vi "loadSRMSummary.vi"(7 "Machine":string, 10 "file path (dialog if empty)":path=path "C:/temp/SRM/S141201869.txt") -> (0 "error out":errorcluster)   [LabVIEW 2012]
uses:
  <vilib>/addons/database/Auxilliary.llb/DB Tools Cursor Type.ctl
  <vilib>/addons/database/Connection.llb/DB Tools Open Connec (Path).vi
  <vilib>/addons/database/Connection.llb/Conn Execute.vi
  <vilib>/addons/database/Recordset.llb/Rec Fetch Integer Data (R).vi
  <vilib>/addons/database/Recordset.llb/Rec Destroy - Connection.vi
  <vilib>/addons/database/NI_Database_API.lvlib
panel:
  out "after substring 2":string
  out "after substring":string
  in  "Cluster 2":T1
  out "array":string[][](array[string])
  out "concatenated string":string
  in  "Cluster":T2
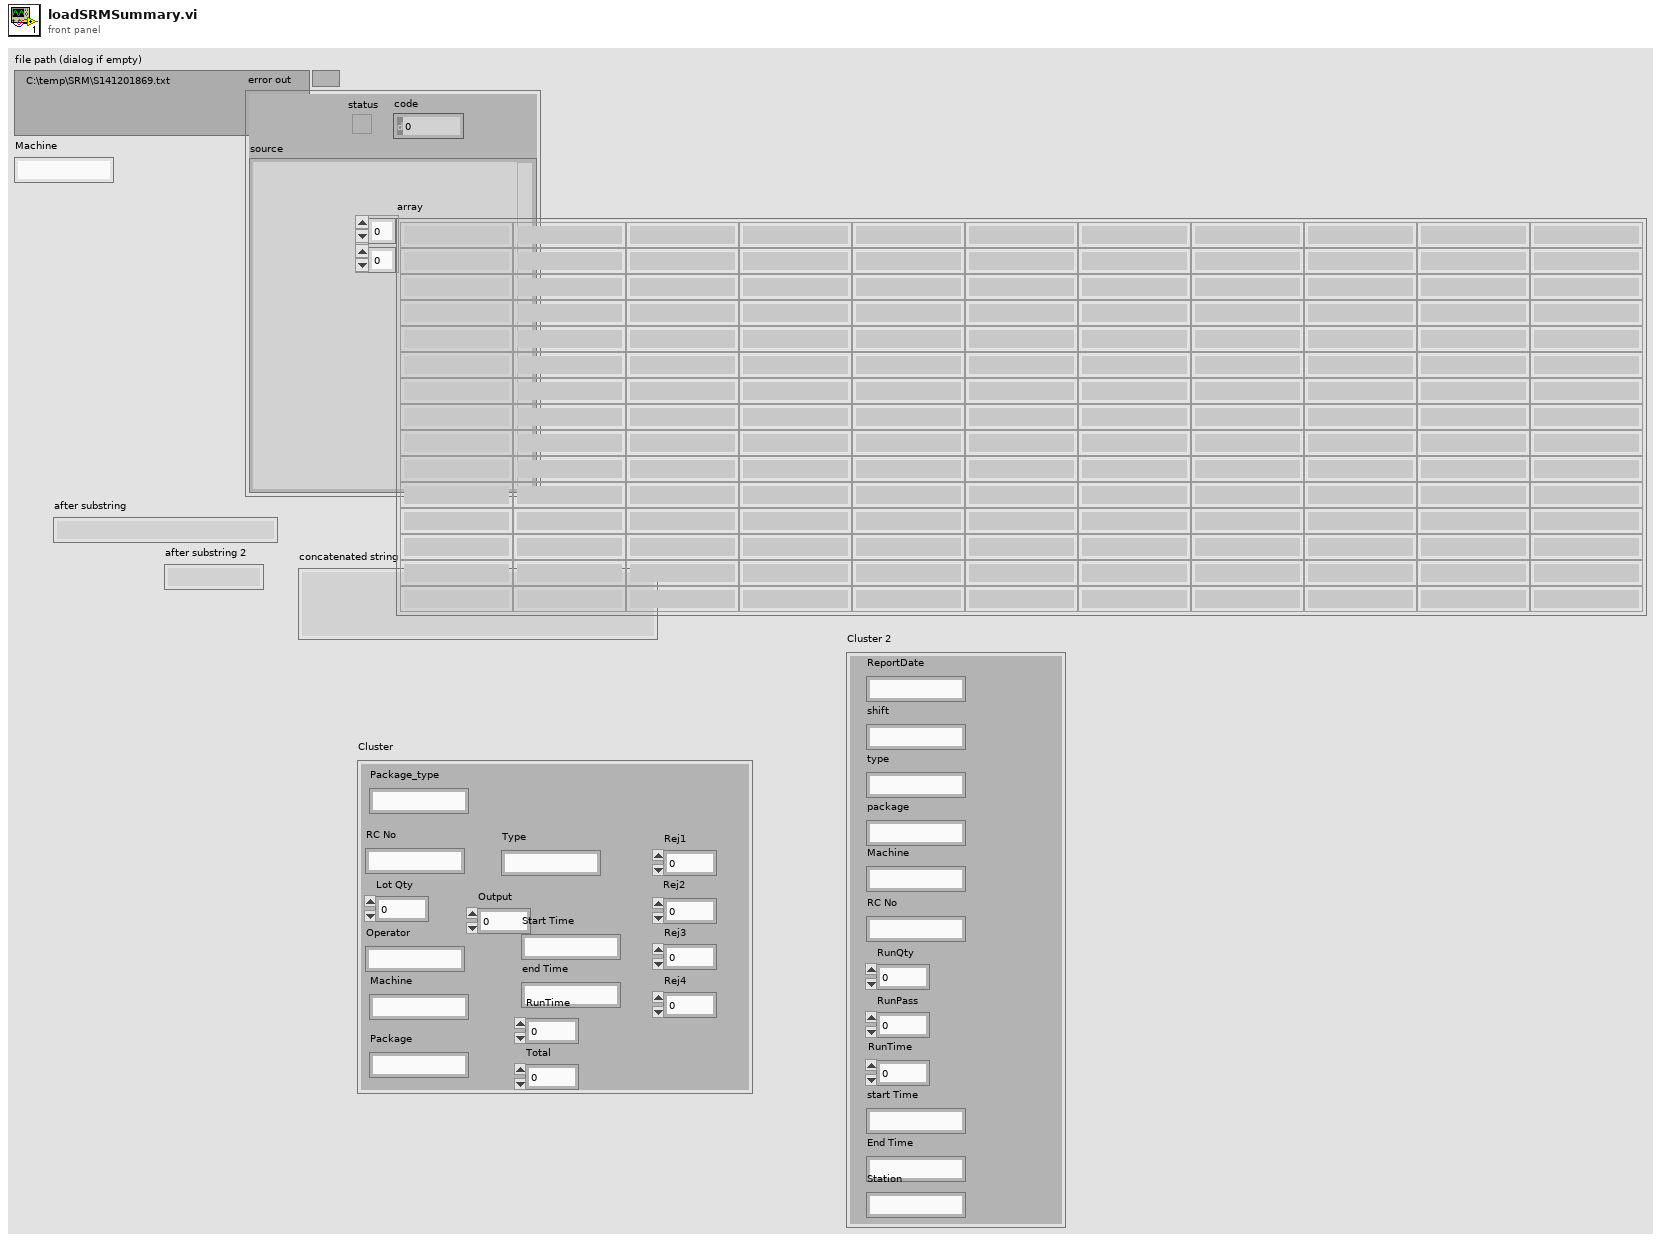
[diagram p1: front panel]
types:
  T1 = cluster{"ReportDate":string, "shift":string, "type":string, "package":string, "Machine":string, "RC No":string, "RunQty":dbl, "RunPass":dbl, "RunTime":dbl, "start Time":string, "End Time":string, "Station":string}
  T2 = cluster{"Package_type":string, "RC No":string, "Lot Qty":dbl, "Operator":string, "Machine":string, "Package":string, "Type":string, "Output":dbl, "Start Time":string, "end Time":string, "RunTime":dbl, "Total":dbl, "Rej1":dbl, "Rej2":dbl, "Rej3":dbl, "Rej4":dbl}
  T3 = typedef "NI_Database_API.lvlib/DB Tools Cursor Type.ctl" = enum16{"forward-only", "keyset", "dynamic", "static"}
  T4 = typedef "NI_Database_API.lvlib/Conn ObjectReference.ctl" = refnum<k1>
  T5 = typedef "NI_Database_API.lvlib/Rec ObjectReference.ctl" = refnum<k1>
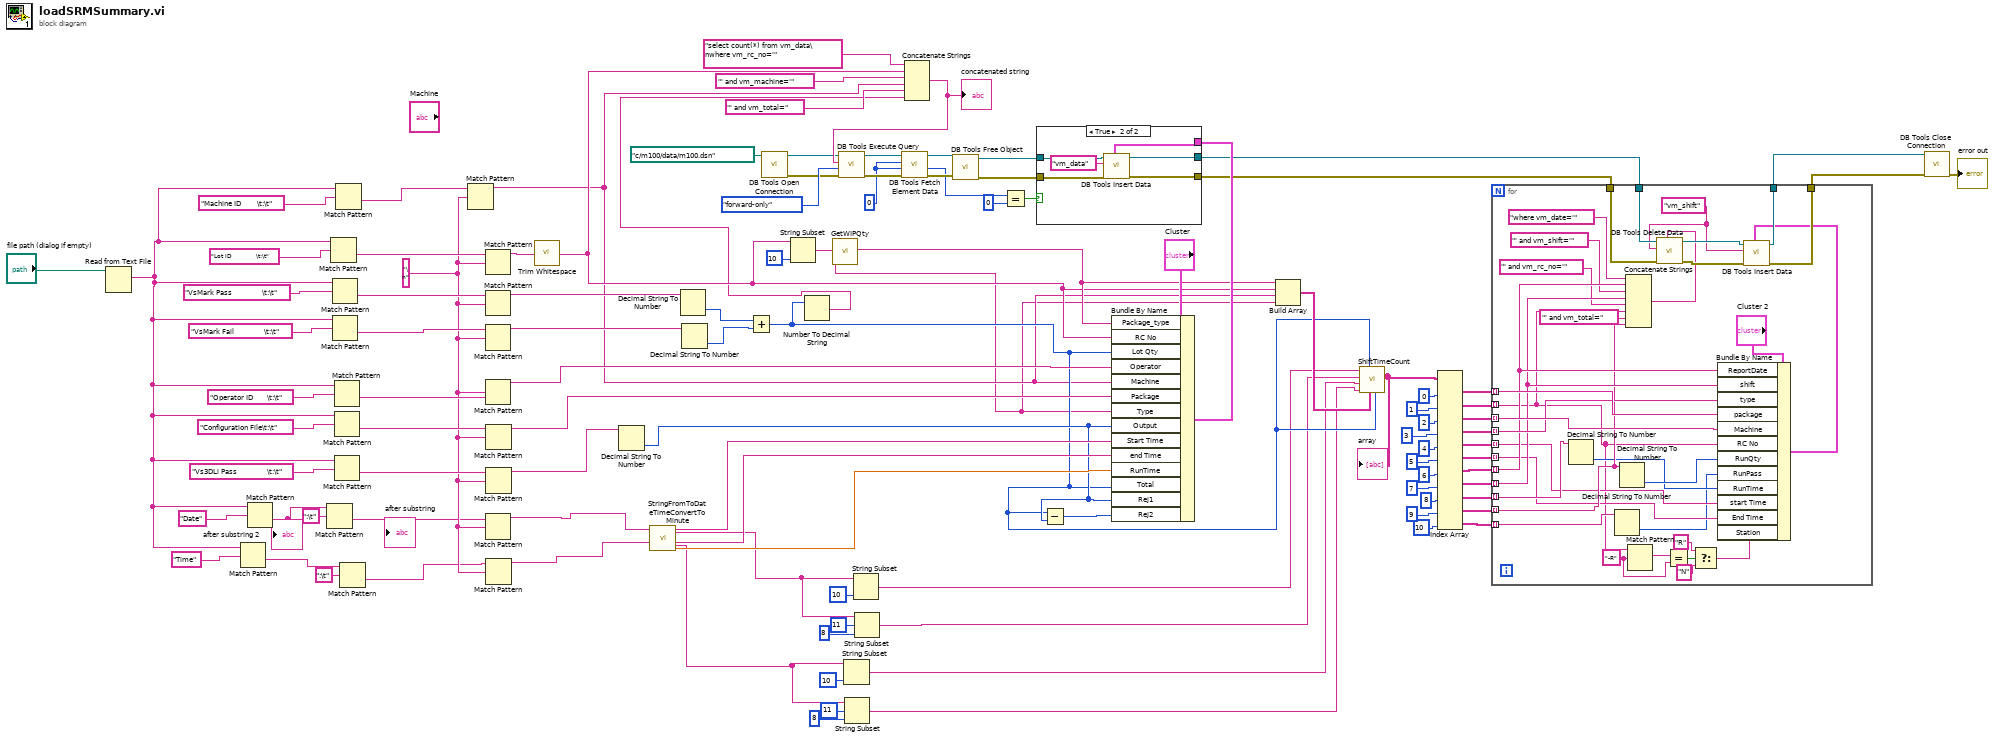
[diagram p0: block diagram]
diagram:
  w84 = 0
  w9 = "\n" ("regular expression")
  n1 = Read from Text File(file (use dialog)="file path (dialog if empty)") -> (text=w11:string)  [unwired: 3 in, 3 out]
  n2 = Match Pattern(string=w11, regular expression="Time") -> (after substring=w3:string)  [unwired: 1 in, 3 out]
  n3 = Match Pattern(string=w11, regular expression="Date") -> (after substring=w6:string)  [unwired: 1 in, 3 out]
  "after substring 2" <- w6
  n4 = Match Pattern(string=w6, regular expression=":\t") -> (after substring=w2:string)  [unwired: 1 in, 3 out]
  "after substring" <- w2
  n5 = Match Pattern(string=w11, regular expression="Lot ID            \t:\t") -> (after substring=w106:string)  [unwired: 1 in, 3 out]
  n6 = Match Pattern(string=w11, regular expression="VsMark Pass               \t:\t") -> (after substring=w105:string)  [unwired: 1 in, 3 out]
  n7 = Match Pattern(string=w11, regular expression="VsMark Fail               \t:\t") -> (after substring=w102:string)  [unwired: 1 in, 3 out]
  n8 = Match Pattern(string=w11, regular expression="Operator ID       \t:\t") -> (after substring=w99:string)  [unwired: 1 in, 3 out]
  n9 = Match Pattern(string=w11, regular expression="Configuration File\t:\t") -> (after substring=w98:string)  [unwired: 1 in, 3 out]
  n10 = Match Pattern(string=w11, regular expression="Vs3DLi Pass               \t:\t") -> (after substring=w96:string)  [unwired: 1 in, 3 out]
  n11 = Match Pattern(string=w11, regular expression="Machine ID        \t:\t") -> (after substring=w10:string)  [unwired: 1 in, 3 out]
  n12 = Match Pattern(string=w3, regular expression=":\t") -> (after substring=w1:string)  [unwired: 1 in, 3 out]
  n13 = Match Pattern(string=w10, regular expression=w9) -> (before substring=w8:string)  [unwired: 1 in, 3 out]
  n14 = Match Pattern(string=w106, regular expression=w9) -> (before substring=w77:string)  [unwired: 1 in, 3 out]
  n15 = Match Pattern(string=w105, regular expression=w9) -> (before substring=w104:string)  [unwired: 1 in, 3 out]
  n16 = Match Pattern(string=w102, regular expression=w9) -> (before substring=w38:string)  [unwired: 1 in, 3 out]
  n17 = Match Pattern(string=w99, regular expression=w9) -> (before substring=w35:string)  [unwired: 1 in, 3 out]
  n18 = Match Pattern(string=w2, regular expression=w9) -> (before substring=w33:string)  [unwired: 1 in, 3 out]
  n19 = Match Pattern(string=w98, regular expression=w9) -> (before substring=w71:string)  [unwired: 1 in, 3 out]
  n20 = Match Pattern(string=w96, regular expression=w9) -> (before substring=w34:string)  [unwired: 1 in, 3 out]
  n21 = Match Pattern(string=w1, regular expression=w9) -> (before substring=w32:string)  [unwired: 1 in, 3 out]
  n22 = call <vilib>:"Trim Whitespace.vi"("string"=w77) -> ("trimmed string"=w67:string)  [unwired: 1 in]
  n23 = Decimal String To Number(string=w34) -> (number=w28:i32)  [unwired: 2 in, 1 out]
  n24 = call "StringFromToDateTimeConvertToMinute.vi"("FromToTime"=w32, "FromToDate"=w33) -> ("Min"=w29:dbl, "End"=w30:string, "Start"=w31:string, "EndMDY"=w15:string, "StartMDY"=w23:string)  [unwired: 5 in]
  n25 = Decimal String To Number(string=w104) -> (number=w37:i32)  [unwired: 2 in, 1 out]
  n26 = Decimal String To Number(string=w38) -> (number=w36:i32)  [unwired: 2 in, 1 out]
  n27 = Add(x=w37, y=w36) -> (x+y=w22:i32)
  n28 = call-poly <vilib>:"DB Tools Open Connection.vi"("connection information"=path "c:/m100/data/m100.dsn") -> ("error out"=w74:errorcluster, "connection reference"=w75:T4)  [unwired: 7 in]
  n29 = String Subset(string=w67, length (rest)=10 ("length (rest)")) -> (substring=w69:string)  [unwired: 1 in]
  n30 = Number To Decimal String(number=w22) -> (decimal integer string=w21:string)  [unwired: 1 in]
  n31 = call "GetWIPQty.vi"("Lotno"=w69) -> ("Package"=w68:string, "loadTool"=w7:string)  [unwired: 2 in, 7 out]
  n32 = String Subset(string=w15, length (rest)=10 ("length (rest)")) -> (substring=w14:string)  [unwired: 1 in]
  n33 = String Subset(string=w15, offset (0)=11, length (rest)=8 ("length (rest)")) -> (substring=w13:string)
  n34 = String Subset(string=w23, length (rest)=10 ("length (rest)")) -> (substring=w20:string)  [unwired: 1 in]
  n35 = String Subset(string=w23, offset (0)=11, length (rest)=8 ("length (rest)")) -> (substring=w19:string)
  n36 = Concatenate Strings("select count(*) from vm_data\nwhere vm_rc_no='" ("SQL query"), w67, "' and vm_machine='" ("string"), w8, "' and vm_total=" ("string"), w21) -> (w76:string)
  "concatenated string" <- w76
  n37 = call-poly <vilib>:"DB Tools Execute Query.vi"("error in (no error)"=w74, "cursor type"=DB_Tools_Cursor_Type."forward-only", "SQL query"=w76, "connection reference"=w75) -> ("error out"=w90:errorcluster, "recordset reference"=w92:T5)  [unwired: 4 in]
  n38 = call-poly <vilib>:"DB Tools Fetch Element Data.vi"("error in (no error)"=w90, "type"=w84, "column index"=w84, "recordset reference"=w92) -> ("error out"=w89:errorcluster, "data"=w83:i32, "recordset reference out"=w91:T5)  [unwired: 3 in]
  n39 = call-poly <vilib>:"DB Tools Free Object.vi"("error in (no error)"=w89, "recordset reference"=w91) -> ("error out"=w79:errorcluster, "connection reference"=w80:T4)  [unwired: 8 in]
  n40 = Equal?(x=w83, y=0) -> (x = y?=w81:bool)
  n41 = Subtract(x=w22, y=w28) -> (x-y=w27:i32)
  n42 = Bundle By Name(cluster="Cluster", "Package_type"=w68, "RC No"=w67, "Lot Qty"=w22, "Operator"=w35, "Machine"=w8, "Package"=w71, "Type"=w7, "Output"=w28, "Start Time"=w31, "end Time"=w30, "RunTime"=w29, "Total"=w22, "Rej1"=w28, "Rej2"=w27) -> (w78:T2)
  n43 = case shown="True" w81 {
    tunnel: w80 -> [w111 w117]
    tunnel: w79 -> [w110 w116]
    tunnel: [w111 w115] -> w44
    tunnel: [w110 w114] -> w43
    tunnel: w78 -> [_ w113]
    frame False {
    }
    frame True {
      n44 = call <vilib>:"DB Tools Insert Data.vi"("data"=w113, "error in (no error)"=w116, "table"="vm_data", "connection reference"=w117) -> ("error out"=w114:errorcluster, "connection reference out"=w115:T4)  [unwired: 6 in]
    }
  }
  n45 = Build Array(w68, w67, w8, w7) -> (w66:string[])
  n46 = call "ShiftTimeCount.vi"("PASS"=w22, "BasicData"=w66, "Qty"=w22, "EndTime 2"=w13, "date string"=w14, "BegTime"=w19, "BegDate"=w20) -> ("array"=w65:string[][])  [unwired: 4 in]
  "array" <- w65
  n47 = Index Array(array=w65, index (col) #1=0 ("disabled index (col)"), index (col) #2=1 ("index (col)"), index (col) #3=2 ("index (col)"), index (col) #4=3 ("index (col)"), index (col) #5=4 ("index (col)"), index (col) #6=5 ("index (col)"), index (col) #7=6 ("index (col)"), index (col) #8=7 ("index (col)"), index (col) #9=8 ("index (col)"), index (col) #10=9 ("index (col)"), index (col) #11=10 ("index (col)")) -> (element #1=w54:string[], element #2=w53:string[], element #3=w52:string[], element #4=w51:string[], element #5=w50:string[], element #6=w49:string[], element #7=w48:string[], element #8=w47:string[], element #9=w46:string[], element #10=w45:string[], element #11=w39:string[])  [unwired: 11 in]
  n48 = for {
    tunnel: w54 -> [w150] mode=indexing
    tunnel: w53 -> [w124] mode=indexing
    tunnel: w52 -> [w149] mode=indexing
    tunnel: w51 -> [w148] mode=indexing
    tunnel: w50 -> [w128] mode=indexing
    tunnel: w49 -> [w129] mode=indexing
    tunnel: w48 -> [w135] mode=indexing
    tunnel: w47 -> [w133] mode=indexing
    tunnel: w46 -> [w147] mode=indexing
    tunnel: w45 -> [w130] mode=indexing
    tunnel: w44 -> [w140]
    tunnel: w43 -> [w139]
    tunnel: [w145] -> w42
    tunnel: [w144] -> w41
    tunnel: w39 -> [w125] mode=indexing
    w122 = "-R" ("regular expression")
    w138 = "vm_shift" ("table")
    n49 = Decimal String To Number(string=w147) -> (number=w127:i32)  [unwired: 2 in, 1 out]
    n50 = Decimal String To Number(string=w125) -> (number=w126:i32)  [unwired: 2 in, 1 out]
    n51 = Decimal String To Number(string=w130) -> (number=w146:i32)  [unwired: 2 in, 1 out]
    n52 = Concatenate Strings("where vm_date='" ("string"), w135, "' and vm_shift='" ("string"), w133, "' and vm_rc_no='" ("string"), w124, "' and vm_total=" ("string"), w130) -> (w137:string)
    n53 = Match Pattern(string=w124, regular expression=w122) -> (match substring=w123:string)  [unwired: 1 in, 3 out]
    n54 = call <vilib>:"DB Tools Delete Data.vi"("condition"=w137, "error in (no error)"=w139, "table"=w138, "connection reference"=w140) -> ("error out"=w141:errorcluster, "connection reference out"=w142:T4)  [unwired: 6 in]
    n55 = Equal?(x=w123, y=w122) -> (x = y?=w121:bool)
    n56 = Select(t="R", s=w121, f="N") -> (s? t:f=w118:string)
    n57 = Bundle By Name(cluster="Cluster 2", "ReportDate"=w135, "shift"=w133, "type"=w148, "package"=w150, "Machine"=w149, "RC No"=w124, "RunQty"=w146, "RunPass"=w126, "RunTime"=w127, "start Time"=w128, "End Time"=w129, "Station"=w118) -> (w143:T1)
    n58 = call <vilib>:"DB Tools Insert Data.vi"("data"=w143, "error in (no error)"=w141, "table"=w138, "connection reference"=w142) -> ("error out"=w144:errorcluster, "connection reference out"=w145:T4)  [unwired: 6 in]
  }
  n59 = call <vilib>:"DB Tools Close Connection.vi"("error in (no error)"=w41, "connection reference"=w42) -> ("error out"=→"error out":errorcluster)  [unwired: 5 in]
